vi "Next Value in Line.vi"(11 "string in":string) -> (0 "value":string, 3 "rest of string":string)   [LabVIEW 2018]
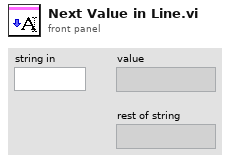
[diagram p1: front panel]
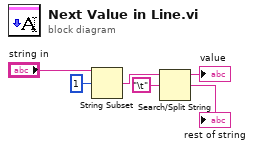
[diagram p0: block diagram]
diagram:
  n1 = String Subset(string="string in", offset (0)=1) -> (substring=w3:string)  [unwired: 1 in]
  n2 = Search/Split String(string=w3, search string/char (-)="\t") -> (substring before match=→"value":string, match + rest of string=→"rest of string":string)  [unwired: 1 in, 1 out]
